vi "programming_split_panels.vi"() -> ()   [LabVIEW 2024]
panel:
  in  "Plots":bool
  out "Waveform Graph":dbl[](graph)
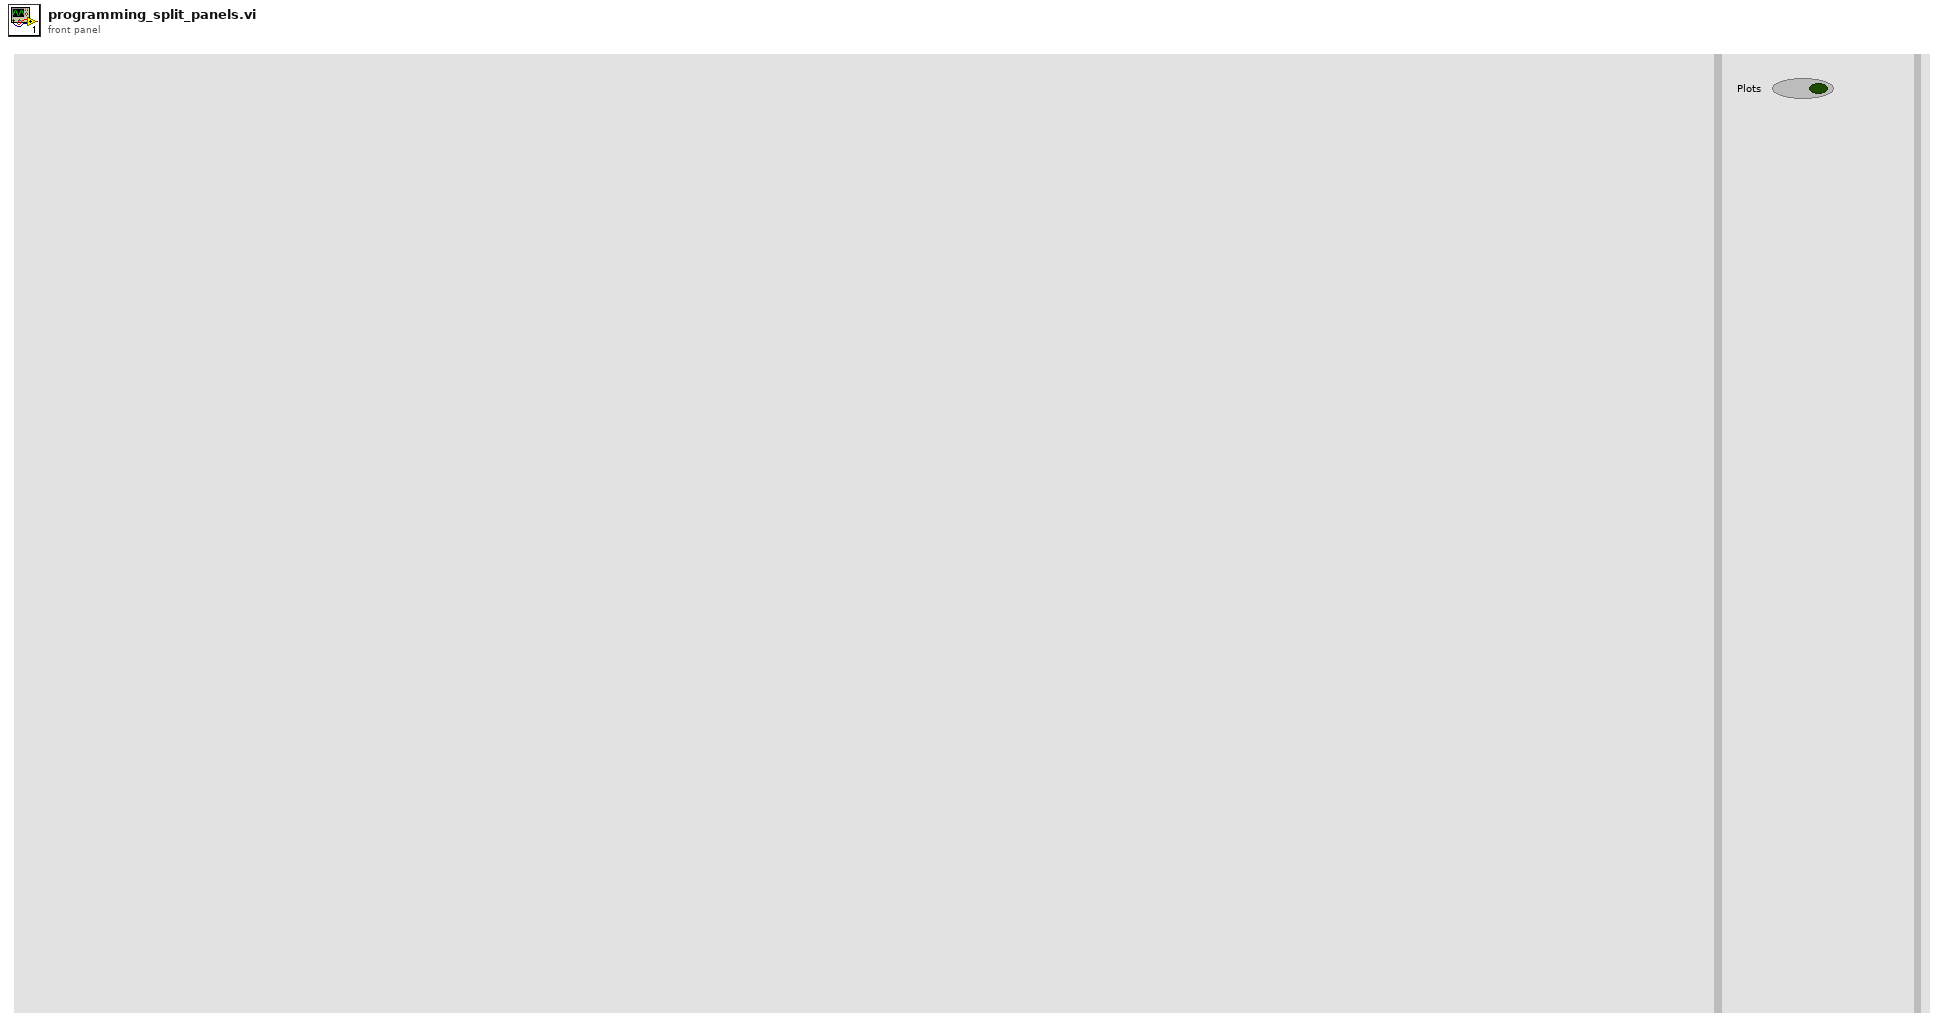
[diagram p1: front panel]
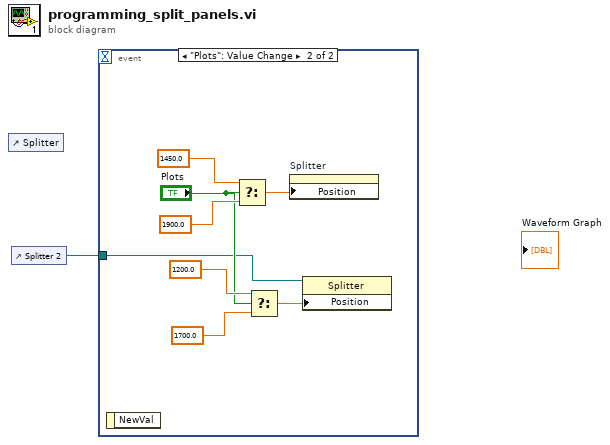
[diagram p0: block diagram]
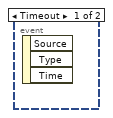
[diagram p2: hidden frame]
diagram:
  n1 = control-ref of="Splitter"() -> ()  [unwired: 1 out]
  n2 = control-ref of="Splitter 2"() -> (w1:refnum<vi>)
  n3 = event shown="[1] \"Plots\": Value Change" {
    selector: _ -> [_ _]
    dyn-events: _ -> [_ _]
    timeout: _ -> [_ _]
    tunnel: w1 -> [_ w2]
    event Timeout {
      n4 = event-data() -> ()  [unwired: 1 in, 3 out]
    }
    event "Plots": Value Change {
      n5 = event-data() -> ()  [unwired: 1 in, 1 out]
      n6 = Select(t=1450.0, s="Plots", f=1900.0) -> (s? t:f=w7:dbl)
      n7 = Select(t=1200.0, s="Plots", f=1700.0) -> (s? t:f=w3:dbl)
      n8 = property on="Splitter" class="Splitter"("Position"=w7) -> ()  [unwired: 2 in, 2 out]
      n9 = property class="Splitter"(reference=w2, "Position"=w3) -> ()  [unwired: 1 in, 2 out]
    }
  }
